vi "Frontend.vi"() -> ()   [LabVIEW 2016]
uses:
  Driver/Old driver/4155C Filename.vi
panel:
  in  "Panel Controls 2":T1={"Emergency Stop"=refnum, "CapGraph Max"=1e-05, "Text/Graph (text=false)"=FALSE} {"CapGraph Max" format="%.2e"}
  in  "Gate 3":T2={"Gate Start"=0.0, "Gate Stop"=2.0, "Gate Step"=1.0, "Gate Compliance"=0.0001, "Range mode"=0, "Range"=6} {"Range" max=11 scale=0.0..11.0; "Range mode" items=["Auto", "Limited", "Fixed"]; "Gate Compliance" min=0.0 max=0.1 format="%^.2e"; "Gate Step" min=-100.0 max=100.0 format="%^.4e"; "Gate Stop" min=-100.0 max=100.0 format="%^.4e"; "Gate Start" min=-100.0 max=100.0 format="%^.4e"}
  in  "Drain 3":T3={"Drain voltage"=0.0, "Drain Compliance"=0.0001, "Range mode"=0, "Range"=6} {"Range" max=11 scale=0.0..11.0; "Range mode" items=["Auto", "Limited", "Fixed"]; "Drain Compliance" min=0.0 max=0.1 format="%^.2e"; "Drain voltage" min=-100.0 max=100.0 format="%^.4e"}
  in  "Timings 2":T4={"hold time (sec)"=0.0, "delay time (sec)"=0.0, "Step Time (0 disables)"=0.0, "C-Step"=0.1, "CInt"=0.1, "IInt"=0.1} {"IInt" min=0.01 max=10.0 format="%.2f"; "CInt" min=0.01 max=10.0 format="%.2f"; "C-Step" min=0.01 max=10.0 format="%.2f"; "Step Time (0 disables)" min=0.0 format="%.2f"; "delay time (sec)" min=0.0 format="%.4f"; "hold time (sec)" min=0.0 format="%.4f"}
  in  "Gate 2":T5={"Gate Start"=0.0, "Gate Stop"=2.0, "Gate Step (linear only)"=1.0, "Gate Compliance"=0.0001, "Gate PComp"=0.0, "Range mode"=0, "Range"=6} {"Range" max=11 scale=0.0..11.0; "Range mode" items=["Auto", "Limited", "Fixed"]; "Gate PComp" format="%^.2e"; "Gate Compliance" format="%^.2e"; "Gate Step (linear only)" format="%^.4e"; "Gate Stop" format="%^.4e"; "Gate Start" format="%^.4e"}
  in  "Drain":T6={"Drain Start"=0.0, "Drain Stop"=2.0, "Drain Compliance"=0.0001, "Drain Step"=1.0, "Drain PComp"=0.0, "Range mode"=0, "Range"=6} {"Range" max=11 scale=0.0..11.0; "Range mode" items=["Auto", "Limited", "Fixed"]; "Drain PComp" format="%^.2e"; "Drain Step" format="%^.4e"; "Drain Compliance" format="%^.2e"; "Drain Stop" format="%^.4e"; "Drain Start" format="%^.4e"}
  in  "Gate":T7={"Gate Start"=0.0, "Gate Stop"=2.0, "Gate Step"=1.0, "Gate Compliance"=0.0001, "Gate PComp"=0.0, "Range mode"=0, "Range"=6} {"Range" max=11 scale=0.0..11.0; "Range mode" items=["Auto", "Limited", "Fixed"]; "Gate PComp" format="%^.2e"; "Gate Compliance" format="%^.2e"; "Gate Step" format="%^.4e"; "Gate Stop" format="%^.4e"; "Gate Start" format="%^.4e"}
  in  "Drain 2":T8={"Drain Start"=0.0, "Drain Stop"=2.0, "Drain Compliance"=0.0001, "Drain Step (linear only)"=1.0, "Drain PComp"=0.0, "Range mode"=0, "Range"=6} {"Range" max=11 scale=0.0..11.0; "Range mode" items=["Auto", "Limited", "Fixed"]; "Drain PComp" format="%^.2e"; "Drain Step (linear only)" format="%^.4e"; "Drain Compliance" format="%^.2e"; "Drain Stop" format="%^.4e"; "Drain Start" format="%^.4e"}
  in  "Timings":T9={"integration time"=0, "Short/Long integration time"=0.00064, "hold time (sec)"=0.0, "delay time (sec)"=0.0, "Step Time (0 disables)"=0.0, "sweep method"=0, "Pulse period"=0.005, "Base voltage"=0.0, "Pulse width"=0.0005} {"Pulse width" min=0.0005 max=0.1 step=0.0001 format="%.4f"; "Base voltage" format="%^.4e"; "Pulse period" min=0.005 max=1.0 step=0.0001 format="%.4f"; "sweep method" items=["Continuous", "Pulsed"]; "Step Time (0 disables)" format="%.2f"; "delay time (sec)" format="%.4f"; "hold time (sec)" format="%.4f"; "Short/Long integration time" format="%^.0e"; "integration time" scale=0.0..2.0}
  in  "Panel controls":T10={"Emergency Stop"=refnum, "OutputGraph Max"=1e-05, "Text/Graph (text=false)"=FALSE} {"OutputGraph Max" format="%.2e"}
  in  "Panel Controls":T11={"Emergency Stop"=refnum, "TransGraph Max"=1e-05, "Text/Graph (text=false)"=FALSE, "TransGraph Min"=1e-05} {"TransGraph Min" format="%.2e"; "TransGraph Max" format="%.2e"}
  in  "Tab Control":enum32{"Characteristics", "Other parameters"}(tab)
  in  "Drain Voltage":dbl min=-100.0 max=100.0 format="%.2f"
  in  "Cap voltage":dbl=0.1 min=0.0 max=10.0 format="%.2f"
  in  "Leak I-time":dbl=0.1 min=0.02 max=2.0 step=0.02 format="%.2f"
  in  "Cap I-time":dbl=0.1 min=0.04 max=400.0 step=0.02 format="%.2f"
  in  "QSCV Start":bool
  in  "Gate: Step 2":dbl=-2.0 format="%.2f"
  in  "Gate: Stop 2":dbl=-60.0 min=-100.0 max=100.0 format="%.2f"
  in  "Gate: Start 2":dbl min=-100.0 max=100.0 format="%.2f"
  in  "sweep method":u16(ring) items=["Continuous", "Pulsed"]
  out "Is":dbl format="%.2e"
  out "Id":dbl format="%.2e"
  out "Ig":dbl format="%.2e"
  in  "Vd":dbl(slide) min=-100.0 max=100.0 step=0.1 scale=-100.0..100.0 scale format="%.1f"
  in  "Vg":dbl(slide) min=-100.0 max=100.0 step=0.1 scale=-100.0..100.0 scale format="%.1f"
  in  "Real time sweep":bool
  in  "Interrupt run":bool
  in  "Running":bool=TRUE
  out "Path":path
  in  "integration time":u32(slide)=1 max=2 step=1 scale=0.0..2.0
  in  "sweep mode":u16(ring)=1 items=["Single", "Double"]
  in  "Transfer Start":bool
  in  "Output Start":bool
  in  "Drain: Step":dbl=1.0 min=-100.0 max=100.0 format="%.2f"
  in  "Drain: Stop":dbl=60.0 min=-100.0 max=100.0 format="%.2f"
  in  "Drain:Start":dbl min=-100.0 max=100.0 format="%.2f"
  in  "Gate: Step":dbl=10.0 min=-100.0 max=100.0 format="%.2f"
  in  "Gate: Stop":dbl=60.0 min=-100.0 max=100.0 format="%.2f"
  in  "Gate: Start":dbl min=-100.0 max=100.0 format="%.2f"
  out "XY Graph":cluster{"Y data in":dbl[], "X data in":dbl[]}[](graph)
  in  "Drain: Compliance":dbl=0.01 min=1e-12 max=0.1 format="%.8f"
  in  "Gate: Compliance":dbl=0.001 min=1e-12 max=0.1 format="%.8f"
  in  "Drain: Step":dbl=-55.0 min=-100.0 max=100.0 format="%.3f"
  in  "Drain: Stop":dbl=-60.0 min=-100.0 max=100.0 format="%.3f"
  in  "Drain:Start":dbl=-5.0 min=-100.0 max=100.0 format="%.3f"
  in  "Gate: Step":dbl=-1.0 min=-100.0 max=100.0 format="%.2f"
  in  "Gate: Stop":dbl=-60.0 min=-100.0 max=100.0 format="%.2f"
  in  "Gate: Start":dbl=10.0 min=-100.0 max=100.0 format="%.2f"
  in  "TransGraph Min":dbl=1e-11 format="%.2e"
  in  "Logfile?":bool
  in  "SMU4":cluster{"on/off":bool, "Voltage":dbl} {"Voltage" min=-100.0 max=100.0 format="%.2f"}
  in  "Pulse width":dbl=0.02 min=0.0005 max=0.1 step=0.0001 format="%.4f"
  in  "Base voltage":dbl min=-100.0 max=100.0 format="%.2f"
  in  "Pulse period":dbl=0.5 min=0.005 max=1.0 step=0.0001 format="%.4f"
  in  "Source/Drain\nRange":u8(slide)=3 max=11 scale=0.0..11.0
  in  "Source/Drain\nRange mode":u16(ring)=1 items=["Auto", "Limited", "Fixed"]
  in  "Gate Range":u8(slide)=3 max=11 scale=0.0..11.0
  in  "Gate Range\nmode":u16(ring)=1 items=["Auto", "Limited", "Fixed"]
  in  "Drain Power Compliance":dbl min=0.0 max=1.0 format="%.2f"
  in  "Gate Power\nCompliance":dbl min=0.0 max=1.0 format="%.2f"
  in  "OutputGraph Max":dbl=0.0001 format="%.2e"
  in  "TransGraph Max":dbl=0.001 format="%.2e"
  in  "SPA Display":bool=TRUE
  in  "Step delay /s":dbl min=0.0 max=1.0 format="%.2f"
  in  "Integration time (long)":dbl=0.32 min=0.04 max=2.0 step=0.02 format="%.2f"
  in  "Integration time (short)":dbl=0.00096 min=8e-05 max=0.00192 step=8e-05 format="%^.0e"
  in  "hold time /s":dbl min=0.0 max=655.35 step=0.01 format="%.2f"
  in  "delay time /s":dbl min=0.0 max=65.535 step=0.0001 format="%.2f"
  in  "Decimal places in header":i8=1
  out "error out":errorcluster
  # "Transfer Characteristics"
  # "V"
  # "V"
  # "V"
  # "Gate"
  # "V"
  # "V"
  # "Drain"
  # "V"
  # "Output Characteristics"
  # "V"
  # "V"
  # "V"
  # "Gate"
  # "V"
  # "V"
  # "Drain"
  # "V"
  # "Quasi Static Capacitance measurement"
  # "V"
  # "V"
  # "V"
  # "Gate"
  # "s"
  # "V"
  # "V"
  # "s"
  # "A"
  # "A"
  # "s"
  # "Pulsed mode settings"
  # "s"
  # "NOTE - THIS OVERRIDES THE COMPLIANCE VALUES!"
  # "A"
  # "A"
  # "Enter max power in Watts (max 1W)"
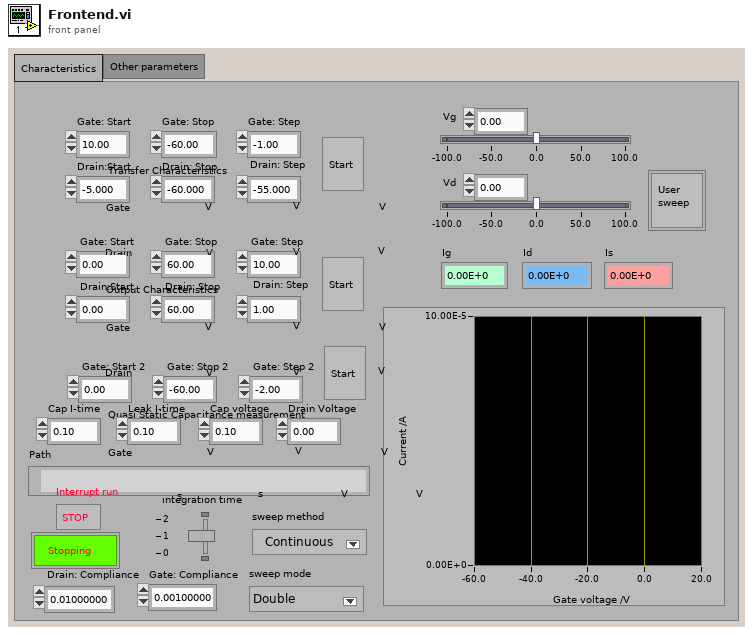
[diagram p1: front panel]
types:
  T1 = cluster{"Emergency Stop":refnum<vi>, "CapGraph Max":dbl, "Text/Graph (text=false)":bool}
  T2 = cluster{"Gate Start":dbl, "Gate Stop":dbl, "Gate Step":dbl, "Gate Compliance":dbl, "Range mode":u16, "Range":u8}
  T3 = cluster{"Drain voltage":dbl, "Drain Compliance":dbl, "Range mode":u16, "Range":u8}
  T4 = cluster{"hold time (sec)":dbl, "delay time (sec)":dbl, "Step Time (0 disables)":dbl, "C-Step":dbl, "CInt":dbl, "IInt":dbl}
  T5 = cluster{"Gate Start":dbl, "Gate Stop":dbl, "Gate Step (linear only)":dbl, "Gate Compliance":dbl, "Gate PComp":dbl, "Range mode":u16, "Range":u8}
  T6 = cluster{"Drain Start":dbl, "Drain Stop":dbl, "Drain Compliance":dbl, "Drain Step":dbl, "Drain PComp":dbl, "Range mode":u16, "Range":u8}
  T7 = cluster{"Gate Start":dbl, "Gate Stop":dbl, "Gate Step":dbl, "Gate Compliance":dbl, "Gate PComp":dbl, "Range mode":u16, "Range":u8}
  T8 = cluster{"Drain Start":dbl, "Drain Stop":dbl, "Drain Compliance":dbl, "Drain Step (linear only)":dbl, "Drain PComp":dbl, "Range mode":u16, "Range":u8}
  T9 = cluster{"integration time":u32, "Short/Long integration time":dbl, "hold time (sec)":dbl, "delay time (sec)":dbl, "Step Time (0 disables)":dbl, "sweep method":u16, "Pulse period":dbl, "Base voltage":dbl, "Pulse width":dbl}
  T10 = cluster{"Emergency Stop":refnum<vi>, "OutputGraph Max":dbl, "Text/Graph (text=false)":bool}
  T11 = cluster{"Emergency Stop":refnum<vi>, "TransGraph Max":dbl, "Text/Graph (text=false)":bool, "TransGraph Min":dbl}
  T12 = cluster{"V2 Start":dbl, "V2 Step":dbl, "Number of points":i32}
  T13 = enum16{"open", "replace", "create", "open or create", "replace or create", "replace or create with confirmation"}
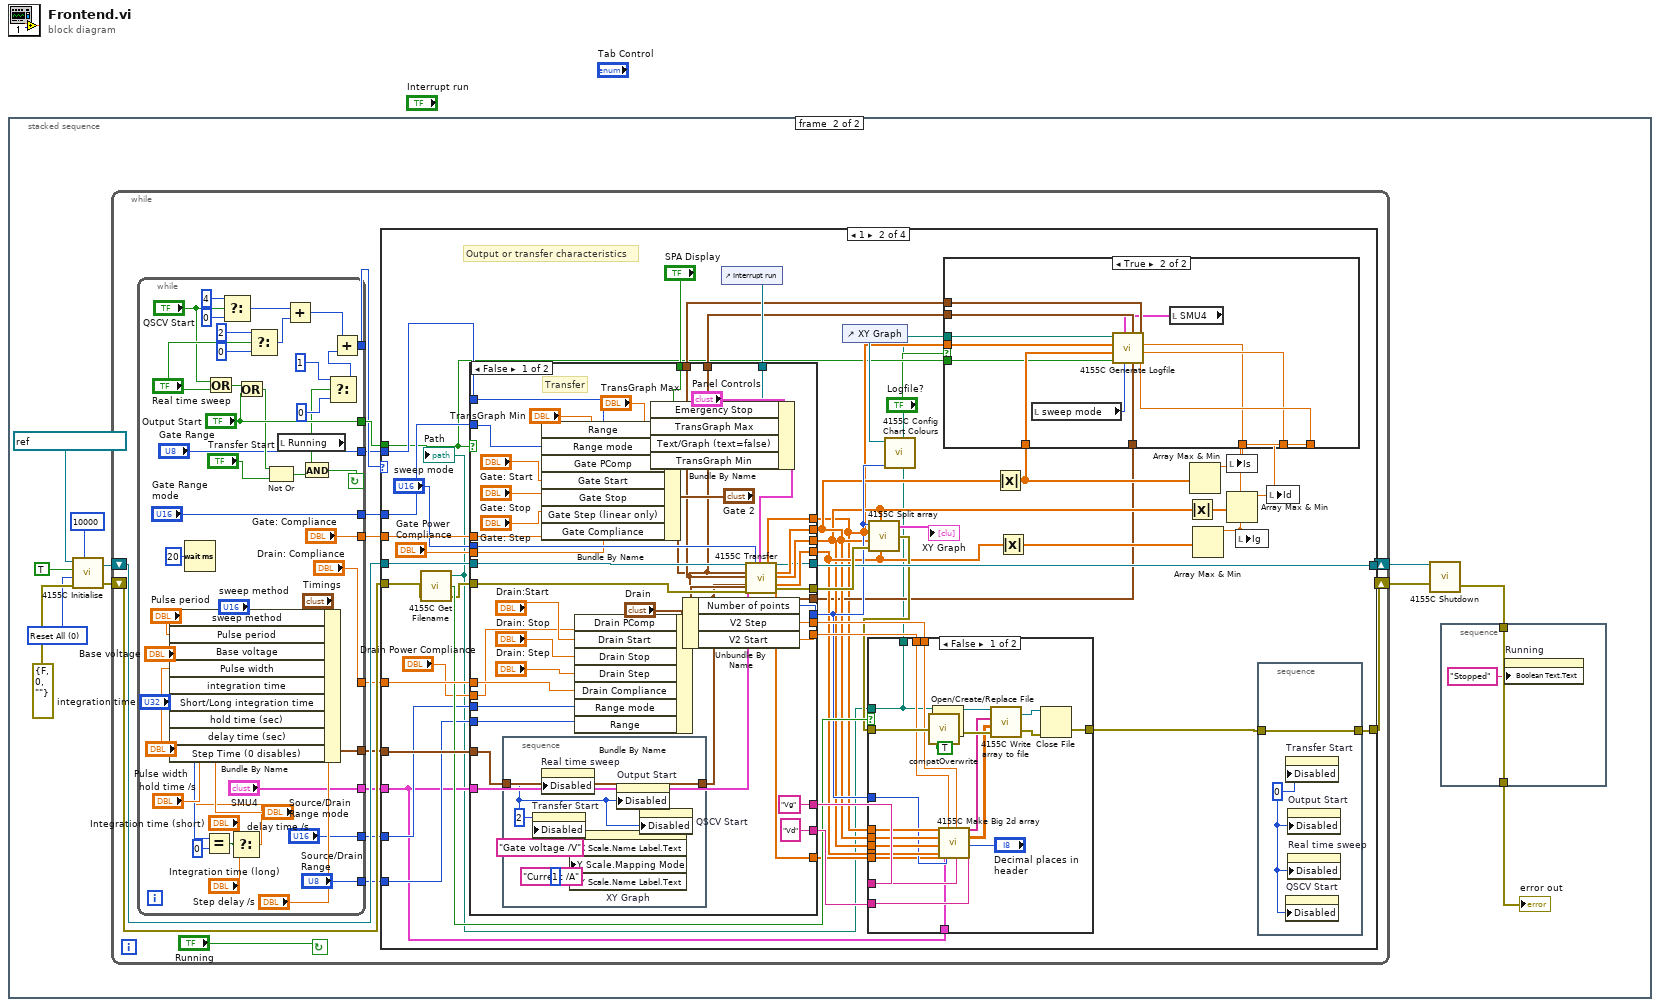
[diagram p0: block diagram]
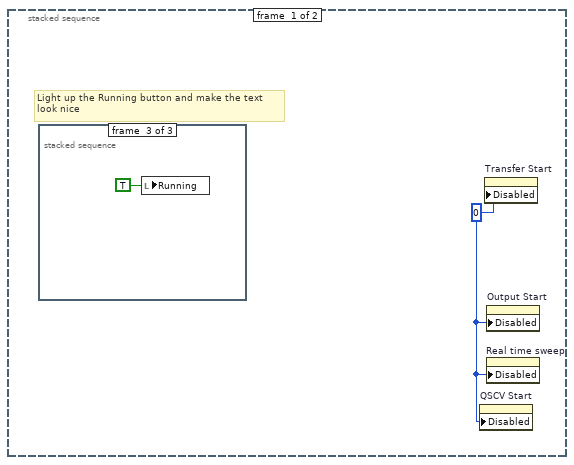
[diagram p2: hidden frame]
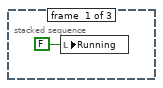
[diagram p3: hidden frame]
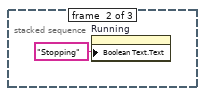
[diagram p4: hidden frame]
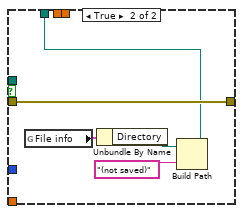
[diagram p7: hidden frame]
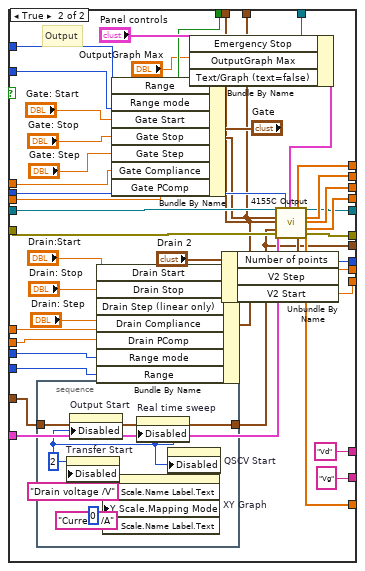
[diagram p8: hidden frame]
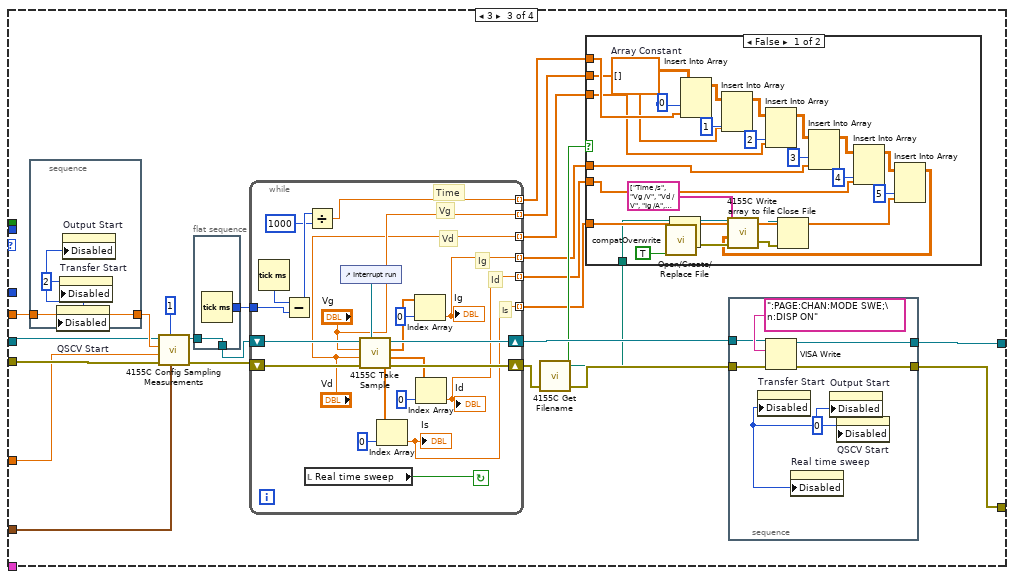
[diagram p9: hidden frame]
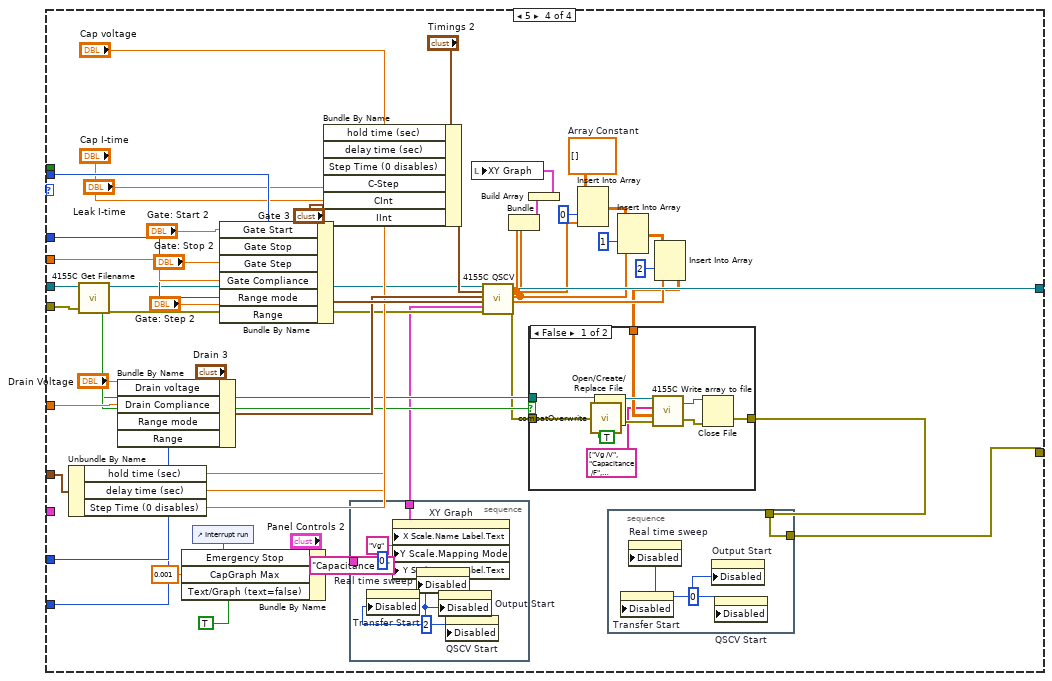
[diagram p11: hidden frame]
diagram:
  n1 = stacked-sequence {
    frame #0 {
      w1 = u8 0 ("Disabled")
      # "Light up the Running button and make the text\nlook nice"
      n2 = stacked-sequence {
        frame #0 {
          n3 = local write "Running"(FALSE ("Running")) -> ()
        }
        frame #1 {
          n4 = property on="Running" class="Bool (strict)"("Boolean Text.Text"="Stopping") -> ()  [unwired: 2 in, 2 out]
        }
        frame #2 {
          (unwired) FALSE ("Running")
          n5 = local write "Running"(TRUE ("Running")) -> ()
        }
      }
      n6 = property on="QSCV Start" class="Bool (strict)"("Disabled"=w1) -> ()  [unwired: 2 in, 2 out]
      n7 = property on="Transfer Start" class="Bool (strict)"("Disabled"=w1) -> ()  [unwired: 2 in, 2 out]
      n8 = property on="Output Start" class="Bool (strict)"("Disabled"=w1) -> ()  [unwired: 2 in, 2 out]
      n9 = property on="Real time sweep" class="Bool (strict)"("Disabled"=w1) -> ()  [unwired: 2 in, 2 out]
    }
    frame #1 {
      w11 = u16 0 items=["Reset All", "Partial reset"] ("Type of reset")
      n10 = call "4155C Initialise.vi"("VISA resource name in"=refnum<visa-resource-name> "GPIB0::14::INSTR", "Reset"=TRUE, "Type of reset"=w11, "error in (no error)"=errorcluster {"status"=FALSE, "code"=0, "source"=""}, "VISA Timeout Value"=u32 10000) -> ("VISA Resource Name out"=w10:refnum<visa-resource-name>, "error out"=w9:errorcluster)
      n11 = while {
        shift-left: w10 -> [w25]
        shift-right: [w27] -> w5
        shift-left: w9 -> [w26]
        shift-right: [w28] -> w6
        stop <- "Running" continue-if-true
        n12 = while {
          tunnel: ["SMU4"] -> w16
          tunnel: ["Gate Range"] -> w17
          tunnel: ["Gate Range\nmode"] -> w18
          tunnel: ["Source/Drain\nRange"] -> w19
          tunnel: ["Source/Drain\nRange mode"] -> w20
          tunnel: ["Drain: Compliance"] -> w21
          tunnel: [w57] -> w22
          tunnel: ["Gate: Compliance"] -> w23
          tunnel: [w63] -> w24
          tunnel: ["Output Start"] -> w29
          stop <- w72 continue-if-true
          n13 = Wait (ms)(milliseconds to wait=u32 20) -> ()  [unwired: 1 out]
          n14 = Equal?(x="integration time", y=u32 0) -> (x = y?=w54:bool)
          n15 = Or(x="QSCV Start", y="Real time sweep") -> (x .or. y?=w42:bool)
          n16 = Select(t=i8 4, s="QSCV Start", f=i8 0) -> (s? t:f=w37:i8)
          n17 = Select(t="Integration time (short)", s=w54, f="Integration time (long)") -> (s? t:f=w51:dbl)
          n18 = Bundle By Name(cluster="Timings", "sweep method"="sweep method", "Pulse period"="Pulse period", "Base voltage"="Base voltage", "Pulse width"="Pulse width", "integration time"="integration time", "Short/Long integration time"=w51, "hold time (sec)"="hold time /s", "delay time (sec)"="delay time /s", "Step Time (0 disables)"="Step delay /s") -> (w57:T9)
          n19 = Or(x=w42, y="Output Start") -> (x .or. y?=w69:bool)
          n20 = Select(t=i8 2, s="Real time sweep", f=i8 0) -> (s? t:f=w38:i8)
          n21 = Not Or(1:"Transfer Start", 2:w69) -> (0:w71:bool)
          n22 = local read "Running"() -> (w66:bool)
          n23 = Add(x=w37, y=w38) -> (x+y=w36:i8)
          n24 = And(x=w66, y=w71) -> (x .and. y?=w72:bool)
          n25 = Select(t=i8 1, s=w66, f=i8 0) -> (s? t:f=w62:i8)
          n26 = Add(x=w36, y=w62) -> (x+y=w63:i8)
        }
        n27 = case shown="1" w24 {
          tunnel: w29 -> [_ w79 _ _]
          tunnel: w22 -> [_ w122 w273 w372]
          tunnel: w23 -> [_ w121 w283 w384]
          tunnel: w21 -> [_ w120 w277 w388]
          tunnel: [w75 w111 w281 w343] -> w28
          tunnel: [w74 w114 w282 w368] -> w27
          tunnel: w26 -> [w75 w105 w279 w364]
          tunnel: w25 -> [w74 w113 w278 w363]
          tunnel: w20 -> [_ w90 _ w381]
          tunnel: w19 -> [_ w89 _ w380]
          tunnel: w18 -> [_ w88 _ w383]
          tunnel: w17 -> [_ w87 _ w382]
          tunnel: w16 -> [_ w85 _ _]
          frame 0, Default {
            # "Someone's deselected the running button so just shutdown..."
          }
          frame 1 {
            # "Output or transfer characteristics"
            n28 = call "4155C Get Filename.vi"("error in (no error)"=w105) -> ("error out"=w104:errorcluster, "cancelled"=w110:bool, "path"=w78:path)  [unwired: 2 in]
            "Path" <- w78
            n29 = control-ref of="Interrupt run"() -> (w106:refnum<vi>)
            n30 = case shown="False" w79 {
              tunnel: w113 -> [w189 w236]
              tunnel: w104 -> [w188 w235]
              tunnel: w122 -> [w192 w241]
              tunnel: w121 -> [w202 w252]
              tunnel: w120 -> [w207 w251]
              tunnel: "sweep mode" -> [w201 w250]
              tunnel: [w200 w249] -> w80
              tunnel: [w199 w248] -> w92
              tunnel: [w198 w247] -> w91
              tunnel: [w197 w246] -> w93
              tunnel: [w196 w245] -> w114
              tunnel: [w195 w244] -> w119
              tunnel: [w171 w220] -> w109
              tunnel: [w172 w219] -> w117
              tunnel: [w173 w218] -> w118
              tunnel: ["Vg" "Vd"] -> w116
              tunnel: ["Vd" "Vg"] -> w115
              tunnel: w106 -> [w186 w234]
              tunnel: "SPA Display" -> [w185 w232]
              tunnel: "Drain Power Compliance" -> [w181 w229]
              tunnel: "Gate Power\nCompliance" -> [w182 w228]
              tunnel: w90 -> [w176 w225]
              tunnel: w89 -> [w175 w224]
              tunnel: w88 -> [w177 w223]
              tunnel: w87 -> [w178 w222]
              tunnel: w85 -> [w170 w217]
              tunnel: [w169 w216] -> w86
              tunnel: [w168 w214] -> w83
              tunnel: [w167 w215] -> w82
              tunnel: [w166 w213] -> w81
              frame False {
                # "Transfer"
                n31 = stacked-sequence {
                  tunnel: w192 -> [w211]
                  tunnel: [w211] -> w166
                  frame #0 {
                    w209 = u8 2 ("Disabled")
                    n32 = property on="Transfer Start" class="Bool (strict)"("Disabled"=w209) -> ()  [unwired: 2 in, 2 out]
                    n33 = property on="Real time sweep" class="Bool (strict)"("Disabled"=w209) -> ()  [unwired: 2 in, 2 out]
                    n34 = property on="XY Graph" class="XYGraph (strict)"("X Scale.Name Label.Text"="Gate voltage /V", "Y Scale.Mapping Mode"=u8 1, "Y Scale.Name Label.Text"="Current /A") -> ()  [unwired: 2 in, 2 out]
                    n35 = property on="Output Start" class="Bool (strict)"("Disabled"=w209) -> ()  [unwired: 2 in, 2 out]
                    n36 = property on="QSCV Start" class="Bool (strict)"("Disabled"=w209) -> ()  [unwired: 2 in, 2 out]
                  }
                }
                n37 = Bundle By Name(cluster="Gate 2", "Range"=w178, "Range mode"=w177, "Gate PComp"=w182, "Gate Start"="Gate: Start", "Gate Stop"="Gate: Stop", "Gate Step (linear only)"="Gate: Step", "Gate Compliance"=w202) -> (w167:T5)
                n38 = Bundle By Name(cluster="Drain", "Drain PComp"=w181, "Drain Start"="Drain:Start", "Drain Stop"="Drain: Stop", "Drain Step"="Drain: Step", "Drain Compliance"=w207, "Range mode"=w176, "Range"=w175) -> (w168:T6)
                n39 = Bundle By Name(cluster="Panel Controls", "Emergency Stop"=w186, "TransGraph Max"="TransGraph Max", "Text/Graph (text=false)"=w185, "TransGraph Min"="TransGraph Min") -> (w183:T11)
                n40 = call "4155C Transfer.vi"("VISA resource name in"=w189, "Gate"=w167, "Drain"=w168, "Timings"=w166, "error in (no error)"=w188, "SMU4"=w170, "sweep mode"=w201, "Panel Controls"=w183) -> ("VG"=w200:dbl[], "Outparams"=w174:T12, "VISA Resource Name out"=w196:refnum<visa-resource-name>, "IS"=w199:dbl[], "ID"=w198:dbl[], "IG"=w197:dbl[], "error out"=w195:errorcluster, "SMU4"=w169:dbl[])  [unwired: 12 in]
                n41 = Unbundle By Name(w174) -> ("Number of points"=w171:i32, "V2 Step"=w172:dbl, "V2 Start"=w173:dbl)
              }
              frame True {
                # "Output"
                n42 = stacked-sequence {
                  tunnel: w241 -> [w258]
                  tunnel: [w258] -> w213
                  frame #0 {
                    w256 = u8 2 ("Disabled")
                    n43 = property on="Transfer Start" class="Bool (strict)"("Disabled"=w256) -> ()  [unwired: 2 in, 2 out]
                    n44 = property on="Output Start" class="Bool (strict)"("Disabled"=w256) -> ()  [unwired: 2 in, 2 out]
                    n45 = property on="XY Graph" class="XYGraph (strict)"("X Scale.Name Label.Text"="Drain voltage /V", "Y Scale.Mapping Mode"=u8 0, "Y Scale.Name Label.Text"="Current /A") -> ()  [unwired: 2 in, 2 out]
                    n46 = property on="Real time sweep" class="Bool (strict)"("Disabled"=w256) -> ()  [unwired: 2 in, 2 out]
                    n47 = property on="QSCV Start" class="Bool (strict)"("Disabled"=w256) -> ()  [unwired: 2 in, 2 out]
                  }
                }
                n48 = Bundle By Name(cluster="Drain 2", "Drain Start"="Drain:Start", "Drain Stop"="Drain: Stop", "Drain Step (linear only)"="Drain: Step", "Drain Compliance"=w251, "Drain PComp"=w229, "Range mode"=w225, "Range"=w224) -> (w214:T8)
                n49 = Bundle By Name(cluster="Gate", "Range"=w222, "Range mode"=w223, "Gate Start"="Gate: Start", "Gate Stop"="Gate: Stop", "Gate Step"="Gate: Step", "Gate Compliance"=w252, "Gate PComp"=w228) -> (w215:T7)
                n50 = Bundle By Name(cluster="Panel controls", "Emergency Stop"=w234, "OutputGraph Max"="OutputGraph Max", "Text/Graph (text=false)"=w232) -> (w230:T10)
                n51 = call "4155C Output.vi"("VISA resource name in"=w236, "Gate"=w215, "Drain"=w214, "Timings"=w213, "error in (no error)"=w235, "SMU4"=w217, "sweep mode"=w250, "Panel controls"=w230) -> ("VD"=w249:dbl[], "Outparams"=w221:T12, "VISA Resource Name out"=w245:refnum<visa-resource-name>, "IS"=w248:dbl[], "ID"=w247:dbl[], "IG"=w246:dbl[], "error out"=w244:errorcluster, "SMU4"=w216:dbl[])  [unwired: 12 in]
                n52 = Unbundle By Name(w221) -> ("Number of points"=w220:i32, "V2 Step"=w219:dbl, "V2 Start"=w218:dbl)
              }
            }
            n53 = control-ref of="XY Graph"() -> (w107:refnum<vi>)
            n54 = call "4155C Split array.vi"("Number of VAR2 steps"=w109, "Y2 data in"=w91, "X data in"=w80, "Y1 data in"=w92, "Y3 data in"=w93, "error in (no error)"=w119) -> ("Array of clusters"=→"XY Graph":cluster{"Y data in":dbl[], "X data in":dbl[]}[], "error out"=w103:errorcluster)  [unwired: 1 in]
            n55 = case shown="False" w110 {
              tunnel: w103 -> [w158 w164]
              tunnel: [w154 w164] -> w112
              tunnel: w78 -> [w138 _]
              tunnel: w109 -> [w148 _]
              tunnel: w91 -> [w150 _]
              tunnel: w80 -> [w152 _]
              tunnel: w92 -> [w151 _]
              tunnel: w93 -> [w149 _]
              tunnel: w118 -> [w142 _]
              tunnel: w117 -> [w143 _]
              tunnel: w116 -> [w147 _]
              tunnel: w115 -> [w146 _]
              tunnel: w86 -> [w140 _]
              tunnel: w85 -> [w139 _]
              tunnel: [w138 w160] -> w76
              frame False {
                n56 = call <vilib>:"compatOverwrite.vi"("overwrite (F)"=TRUE) -> ("overwrite?"=w137:T13)
                n57 = Open/Create/Replace File(file path (use dialog)=w138, error in=w158, operation (0:open)=w137) -> (refnum out=w156:refnum<file>, error out=w157:errorcluster)  [unwired: 3 in, 1 out]
                n58 = call "4155C Make Big 2d array.vi"("1D Var1"=w152, "1d IS"=w151, "1d ID"=w150, "1d IG"=w149, "1d SMU4"=w140, "SMU4"=w139, "VAR2 START"=w142, "Number of VAR2 steps"=w148, "VAR2 STEP"=w143, "VAR1 Name"=w147, "Decimal places in header"="Decimal places in header", "VAR2 Name"=w146) -> ("Header array"=w144:string[], "Data array"=w145:dbl[][])  [unwired: 14 in]
                n59 = call "4155C Write array to file.vi"("Byte Stream File Refnum"=w156, "Header"=w144, "Data Array"=w145, "error in (no error)"=w157) -> ("dup refnum"=w153:refnum<file>, "error out"=w155:errorcluster)  [unwired: 1 in]
                n60 = Close File(refnum=w153, error in=w155) -> (error out=w154:errorcluster)  [unwired: 1 out]
              }
              frame True {
                n61 = global read "4155C Filename.vi" "File info"() -> (w163:cluster{"Filename":string, "Directory":path})
                n62 = Unbundle By Name(w163) -> ("Directory"=w162:path)
                n63 = Build Path(base path=w162, name or relative path="(not saved)") -> (appended path=w160:path)
              }
            }
            n64 = call "4155C Config Chart Colours.vi"("Numeric"=w109, "XY Graph 2"=w107) -> ()  [unwired: 6 in]
            n65 = Absolute Value(x=w92) -> (abs(x)=w84:dbl[])
            n66 = Absolute Value(x=w93) -> (abs(x)=w98:dbl[])
            n67 = Absolute Value(x=w91) -> (abs(x)=w97:dbl[])
            n68 = Array Max & Min(array=w84) -> (max value=w95:dbl)  [unwired: 3 out]
            n69 = Array Max & Min(array=w98) -> (max value=w96:dbl)  [unwired: 3 out]
            n70 = local write "Is"(w95) -> ()
            n71 = Array Max & Min(array=w97) -> (max value=w94:dbl)  [unwired: 3 out]
            n72 = case shown="True" "Logfile?" {
              tunnel: w84 -> [_ w131]
              tunnel: w95 -> [_ w127]
              tunnel: w94 -> [_ w128]
              tunnel: w96 -> [_ w129]
              tunnel: w83 -> [_ w134]
              tunnel: w82 -> [_ w133]
              tunnel: w81 -> [_ w132]
              tunnel: w80 -> [_ w130]
              tunnel: w76 -> [_ w124]
              tunnel: w79 -> [_ w123]
              frame False {
              }
              frame True {
                n73 = local read "sweep mode"() -> (w125:u16)
                n74 = local read "SMU4"() -> (w126:cluster{"on/off":bool, "Voltage":dbl})
                n75 = call "4155C Generate Logfile.vi"("Ig"=w129, "Id"=w128, "Is"=w127, "Drain"=w134, "Timings"=w132, "Gate"=w133, "sweep mode"=w125, "SMU4"=w126, "Output?"=w123, "Input I"=w131, "VG"=w130, "Path"=w124) -> ()
              }
            }
            n76 = local write "Ig"(w96) -> ()
            n77 = stacked-sequence {
              tunnel: w112 -> [w136]
              tunnel: [w136] -> w111
              frame #0 {
                w135 = u8 0 ("Disabled")
                n78 = property on="Transfer Start" class="Bool (strict)"("Disabled"=w135) -> ()  [unwired: 2 in, 2 out]
                n79 = property on="QSCV Start" class="Bool (strict)"("Disabled"=w135) -> ()  [unwired: 2 in, 2 out]
                n80 = property on="Output Start" class="Bool (strict)"("Disabled"=w135) -> ()  [unwired: 2 in, 2 out]
                n81 = property on="Real time sweep" class="Bool (strict)"("Disabled"=w135) -> ()  [unwired: 2 in, 2 out]
              }
            }
            n82 = local write "Id"(w94) -> ()
          }
          frame 3 {
            n83 = stacked-sequence {
              tunnel: w283 -> [w342]
              tunnel: [w342] -> w280
              frame #0 {
                w341 = u8 2 ("Disabled")
                n84 = property on="QSCV Start" class="Bool (strict)"("Disabled"=w341) -> ()  [unwired: 2 in, 2 out]
                n85 = property on="Transfer Start" class="Bool (strict)"("Disabled"=w341) -> ()  [unwired: 2 in, 2 out]
                n86 = property on="Output Start" class="Bool (strict)"("Disabled"=w341) -> ()  [unwired: 2 in, 2 out]
              }
            }
            n87 = call "4155C Config Sampling Measurements.vi"("Timings"=w273, "Num Points"=i16 1, "error in (no error)"=w279, "Drain Compliance"=w277, "Gate Compliance"=w280, "VISA session"=w278) -> ("error out"=w275:errorcluster, "dup VISA resource name"=w271:refnum<visa-resource-name>)  [unwired: 4 in]
            n88 = flat-sequence {
              tunnel: [w312] -> w272
              tunnel: w271 -> [w312]
              tunnel: [w311] -> w270
              frame #0 {
                n89 = Tick Count (ms)() -> (millisecond timer value=w311:u32)
              }
            }
            n90 = while {
              shift-left: w275 -> [w332]
              shift-right: [w331] -> w269
              shift-left: w272 -> [w333]
              shift-right: [w330] -> w276
              tunnel: ["Vg"] -> w264 mode=indexing
              tunnel: ["Vd"] -> w263 mode=indexing
              tunnel: [w320] -> w262 mode=indexing
              tunnel: [w319] -> w261 mode=indexing
              tunnel: [w318] -> w260 mode=indexing
              tunnel: w270 -> [w316]
              tunnel: [w313] -> w265 mode=indexing
              stop <- w334 continue-if-true
              # "Is"
              # "Id"
              # "Ig"
              # "Vd"
              # "Vg"
              # "Time"
              n91 = Tick Count (ms)() -> (millisecond timer value=w317:u32)
              n92 = Subtract(x=w317, y=w316) -> (x-y=w315:u32)
              n93 = local read "Real time sweep"() -> (w334:bool)
              n94 = Divide(x=w315, y=u32 1000) -> (x/y=w313:dbl)
              n95 = control-ref of="Interrupt run"() -> (w329:refnum<vi>)
              n96 = call "4155C Take Sample.vi"("Emergency Stop"=w329, "error in (no error)"=w332, "Vd"="Vd", "Vg"="Vg", "VISA resource name in"=w333) -> ("error out"=w331:errorcluster, "Id"=w325:dbl[], "Ig"=w323:dbl[], "VISA Resource Name out"=w330:refnum<visa-resource-name>, "Is"=w327:dbl[])  [unwired: 1 in, 1 out]
              n97 = Index Array(array=w327, index=0 ("Index")) -> (element=w318:dbl)
              "Is" <- w318
              n98 = Index Array(array=w323, index=0 ("Index")) -> (element=w320:dbl)
              "Ig" <- w320
              n99 = Index Array(array=w325, index=0 ("Index")) -> (element=w319:dbl)
              "Id" <- w319
            }
            n100 = call "4155C Get Filename.vi"("error in (no error)"=w269) -> ("error out"=w268:errorcluster, "cancelled"=w267:bool, "path"=w266:path)  [unwired: 2 in]
            n101 = case shown="False" w267 {
              tunnel: w266 -> [w291 _]
              tunnel: w265 -> [w308 _]
              tunnel: w264 -> [w299 _]
              tunnel: w263 -> [w298 _]
              tunnel: w262 -> [w297 _]
              tunnel: w261 -> [w296 _]
              tunnel: w260 -> [w293 _]
              frame False {
                w310 = dbl[][] []  # Array Constant
                n102 = call <vilib>:"compatOverwrite.vi"("overwrite (F)"=TRUE) -> ("overwrite?"=w284:T13)
                n103 = Open/Create/Replace File(file path (use dialog)=w291, operation (0:open)=w284) -> (refnum out=w289:refnum<file>, error out=w290:errorcluster)  [unwired: 4 in, 1 out]
                n104 = Insert Into Array(array=w310, index (col)=0 ("Disabled Index (col)"), new element=w308) -> (w307:dbl[][])  [unwired: 1 in]
                n105 = Insert Into Array(array=w307, index (col)=1 ("disabled index (col)"), new element=w299) -> (w306:dbl[][])  [unwired: 1 in]
                n106 = Insert Into Array(array=w306, index (col)=2 ("disabled index (col)"), new element=w298) -> (w305:dbl[][])  [unwired: 1 in]
                n107 = Insert Into Array(array=w305, index (col)=3 ("disabled index (col)"), new element=w297) -> (w304:dbl[][])  [unwired: 1 in]
                n108 = Insert Into Array(array=w304, index (col)=4 ("disabled index (col)"), new element=w296) -> (w295:dbl[][])  [unwired: 1 in]
                n109 = Insert Into Array(array=w295, index (col)=5 ("disabled index (col)"), new element=w293) -> (w287:dbl[][])  [unwired: 1 in]
                n110 = call "4155C Write array to file.vi"("Byte Stream File Refnum"=w289, "Header"=string[] ["Time /s", "Vg /V", "Vd /V", "Ig /A", "Id /A", "Is /A"], "Data Array"=w287, "error in (no error)"=w290) -> ("dup refnum"=w288:refnum<file>, "error out"=w292:errorcluster)  [unwired: 1 in]
                n111 = Close File(refnum=w288, error in=w292) -> ()  [unwired: 2 out]
              }
              frame True {
              }
            }
            n112 = stacked-sequence {
              tunnel: [w337] -> w282
              tunnel: [w336] -> w281
              tunnel: w276 -> [w339]
              tunnel: w268 -> [w338]
              frame #0 {
                w335 = u8 0 ("Disabled")
                n113 = property on="Transfer Start" class="Bool (strict)"("Disabled"=w335) -> ()  [unwired: 2 in, 2 out]
                n114 = VISA Write(VISA resource name=w339, write buffer=":PAGE:CHAN:MODE SWE;\n:DISP ON" ("write buffer (\"\")"), error in (no error)=w338) -> (VISA resource name out=w337:refnum<visa-resource-name>, error out=w336:errorcluster)  [unwired: 1 out]
                n115 = property on="Real time sweep" class="Bool (strict)"("Disabled"=w335) -> ()  [unwired: 2 in, 2 out]
                n116 = property on="Output Start" class="Bool (strict)"("Disabled"=w335) -> ()  [unwired: 2 in, 2 out]
                n117 = property on="QSCV Start" class="Bool (strict)"("Disabled"=w335) -> ()  [unwired: 2 in, 2 out]
              }
            }
          }
          frame 5 {
            w358 = dbl[][] []  # Array Constant
            n118 = Unbundle By Name(w372) -> ("hold time (sec)"=w369:dbl, "delay time (sec)"=w370:dbl, "Step Time (0 disables)"=w371:dbl)
            n119 = call "4155C Get Filename.vi"("error in (no error)"=w364) -> ("error out"=w362:errorcluster, "cancelled"=w361:bool, "path"=w360:path)  [unwired: 2 in]
            n120 = Bundle By Name(cluster="Drain 3", "Drain voltage"="Drain Voltage", "Drain Compliance"=w388, "Range mode"=w381, "Range"=w380) -> (w386:T3)
            n121 = control-ref of="Interrupt run"() -> (w367:refnum<vi>)
            n122 = Bundle By Name(cluster="Panel Controls 2", "Emergency Stop"=w367, "CapGraph Max"=0.001, "Text/Graph (text=false)"=TRUE) -> (w345:T1)
            n123 = Bundle By Name(cluster="Gate 3", "Gate Start"="Gate: Start 2", "Gate Stop"="Gate: Stop 2", "Gate Step"="Gate: Step 2", "Gate Compliance"=w384, "Range mode"=w383, "Range"=w382) -> (w387:T2)
            n124 = Bundle By Name(cluster="Timings 2", "hold time (sec)"=w369, "delay time (sec)"=w370, "Step Time (0 disables)"=w371, "C-Step"="Cap voltage", "CInt"="Cap I-time", "IInt"="Leak I-time") -> (w385:T4)
            n125 = stacked-sequence {
              tunnel: w345 -> [w399]
              tunnel: [w399] -> w346
              frame #0 {
                w398 = u8 2 ("Disabled")
                n126 = property on="Transfer Start" class="Bool (strict)"("Disabled"=w398) -> ()  [unwired: 2 in, 2 out]
                n127 = property on="XY Graph" class="XYGraph (strict)"("X Scale.Name Label.Text"="Vg", "Y Scale.Mapping Mode"=u8 0, "Y Scale.Name Label.Text"="Capacitance /F") -> ()  [unwired: 2 in, 2 out]
                n128 = property on="Real time sweep" class="Bool (strict)"("Disabled"=w398) -> ()  [unwired: 2 in, 2 out]
                n129 = property on="Output Start" class="Bool (strict)"("Disabled"=w398) -> ()  [unwired: 2 in, 2 out]
                n130 = property on="QSCV Start" class="Bool (strict)"("Disabled"=w398) -> ()  [unwired: 2 in, 2 out]
              }
            }
            n131 = call "4155C QSCV.vi"("VISA resource name in"=w363, "Timings"=w385, "Drain"=w386, "Gate"=w387, "Panel Controls"=w346, "error in (no error)"=w362) -> ("VISA Resource Name out"=w368:refnum<visa-resource-name>, "VG"=w350:dbl[], "Cap"=w349:dbl[], "Leak"=w352:dbl[], "error out"=w359:errorcluster)  [unwired: 8 in, 1 out]
            n132 = Bundle("VG"=w350, "Cap"=w349) -> (w348:cluster{"VG":dbl[], "Cap":dbl[]})  [unwired: 1 in]
            n133 = Build Array(w348) -> (w347:cluster{"VG":dbl[], "Cap":dbl[]}[])
            n134 = local write "XY Graph"(w347) -> ()
            n135 = Insert Into Array(array=w358, index (col)=0 ("Disabled Index (col)"), new element=w350) -> (w356:dbl[][])  [unwired: 1 in]
            n136 = Insert Into Array(array=w356, index (col)=1 ("Disabled Index (col)"), new element=w349) -> (w355:dbl[][])  [unwired: 1 in]
            n137 = Insert Into Array(array=w355, index (col)=2 ("Disabled Index (col)"), new element=w352) -> (w351:dbl[][])  [unwired: 1 in]
            n138 = case shown="False" w361 {
              tunnel: w359 -> [w409 w411]
              tunnel: [w404 w411] -> w344
              tunnel: w360 -> [w408 _]
              tunnel: w351 -> [w402 _]
              frame False {
                n139 = call <vilib>:"compatOverwrite.vi"("overwrite (F)"=TRUE) -> ("overwrite?"=w400:T13)
                n140 = Open/Create/Replace File(file path (use dialog)=w408, error in=w409, operation (0:open)=w400) -> (refnum out=w406:refnum<file>, error out=w407:errorcluster)  [unwired: 3 in, 1 out]
                n141 = call "4155C Write array to file.vi"("Byte Stream File Refnum"=w406, "Header"=string[] ["Vg /V", "Capacitance /F", "Leakage current /A"], "Data Array"=w402, "error in (no error)"=w407) -> ("dup refnum"=w403:refnum<file>, "error out"=w405:errorcluster)  [unwired: 1 in]
                n142 = Close File(refnum=w403, error in=w405) -> (error out=w404:errorcluster)  [unwired: 1 out]
              }
              frame True {
              }
            }
            n143 = stacked-sequence {
              tunnel: w344 -> [w394]
              tunnel: [w394] -> w343
              frame #0 {
                w393 = u8 0 ("Disabled")
                n144 = property on="Transfer Start" class="Bool (strict)"("Disabled"=w393) -> ()  [unwired: 2 in, 2 out]
                n145 = property on="Real time sweep" class="Bool (strict)"("Disabled"=w393) -> ()  [unwired: 2 in, 2 out]
                n146 = property on="Output Start" class="Bool (strict)"("Disabled"=w393) -> ()  [unwired: 2 in, 2 out]
                n147 = property on="QSCV Start" class="Bool (strict)"("Disabled"=w393) -> ()  [unwired: 2 in, 2 out]
              }
            }
          }
        }
      }
      n148 = call "4155C Shutdown.vi"("VISA resource name in"=w5, "error in (no error)"=w6) -> ("error out"=w8:errorcluster)  [unwired: 4 in]
      n149 = stacked-sequence {
        tunnel: w8 -> [w413]
        tunnel: [w413] -> w7
        frame #0 {
          n150 = property on="Running" class="Bool (strict)"("Boolean Text.Text"="Stopped") -> ()  [unwired: 2 in, 2 out]
        }
      }
      "error out" <- w7
    }
  }
